vi "Default or Users Font, Leading,Alignment, ASCII or Unicode.vi"(0 "PDF Report":refnum<class "PDF Report Class.lvclass">, 5 "Font":T5={"Name"="", "Size"=-1.0, "Color"=0, "Style"={"Bold"=FALSE, "Italic"=FALSE, "Underline"=FALSE, "Strikeout"=FALSE}, "Type"={"Type&direction"=enum."Select", "Embedded"=FALSE, "Encoding"=""}}, 9 "Paragraphe cluster":T1, 11 "error in (no error)":errorcluster) -> (4 "PDF Report duplicate":refnum<class "PDF Report Class.lvclass">, 6 "Leading":T4=18.0, 8 "Font Ref":refnum<k24>, 10 "Close Font Ref":bool=TRUE, 14 "Aligment":string="JUSTIFY", 15 "error out":errorcluster)   [LabVIEW 2019, in "Exaprom PDF.lvlib"]
doc: "Version 1.0\nDeveloped by Jean-Marc Simard\nCopyright © 2010, Exaprom Inc.\nAll rights reserved.\nLicense: BSD\n\nWith iTextSharp 4.1.6 (http://itextsharp.sourceforge.net)\nunder Mozilla Public License Version 1.1\n(http://www.mozilla.org/MPL/MPL-1.1.html)"
uses:
  LV Class/PDF Report Class/PDF Report Class.lvclass
  Controls/Font Controls/Font complete cluster.ctl
  Controls/Font Controls/Font size.ctl
  Controls/Font Controls/Font color.ctl
  Controls/Font Controls/Type and encoding.ctl
  Controls/Text Controls/Unicode/Type and run direction.ctl
  C:/work/niobrara_lv/labview pdf writer fixing/DLL/itextsharp.dll
  DLL/itextsharp.dll
  Controls/Initialization Controls/Defaut Paragraphe and Line Spacing.ctl
  Controls/Text Controls/Texte alignement.ctl
  Controls/Text Controls/Line spacing.ctl
  Exaprom PDF.lvlib
  LV Class/Fonts Class/Font Class.lvclass
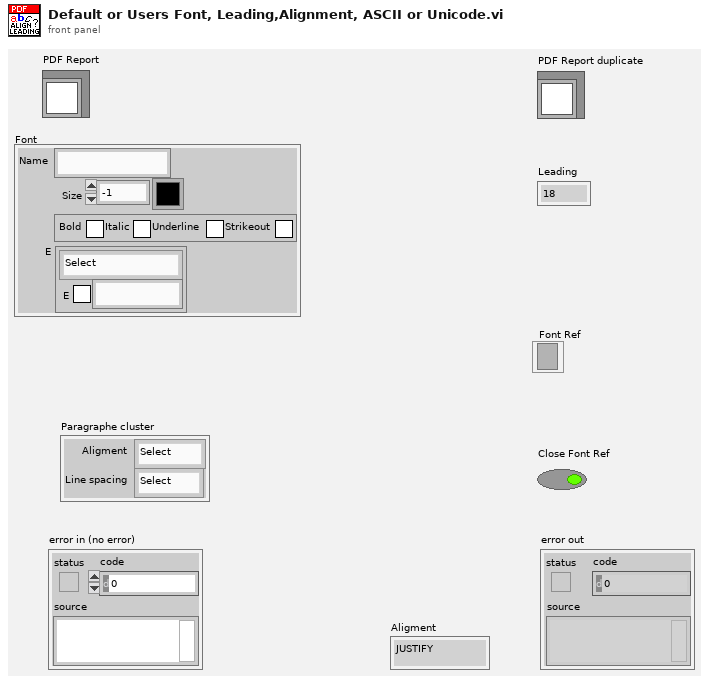
[diagram p1: front panel]
types:
  T1 = typedef "Exaprom PDF.lvlib/Defaut Paragraphe and Line Spacing.ctl" = cluster{" Aligment":T2, "Line spacing":T3}
  T2 = typedef "Exaprom PDF.lvlib/Texte alignement.ctl" = enum16{"Select", "CENTER", "JUSTIFY", "LEFT", "RIGHT"}
  T3 = typedef "Exaprom PDF.lvlib/Line spacing.ctl" = enum16{"Select", "1.0", "1.5", "2.0"}
  T4 = typedef "Exaprom PDF.lvlib/Font size.ctl" = sgl
  T5 = typedef "Exaprom PDF.lvlib/Font complete cluster.ctl" = cluster{"Name":string, "Size":T4, "Color":T6, "Style":cluster{"Bold":bool, "Italic":bool, "Underline":bool, "Strikeout":bool}, "Type":T7}
  T6 = typedef "Exaprom PDF.lvlib/Font color.ctl" = u32
  T7 = typedef "Exaprom PDF.lvlib/Type and encoding.ctl" = cluster{"Type&direction":T8, "Embedded":bool, "Encoding":string}
  T8 = typedef "Exaprom PDF.lvlib/Type and run direction.ctl" = enum16{"Select", "ASCII", "UTF-16", "UTF-16 (default)", "UTF-16 (LTR)", "UTF-16 (RTL)"}
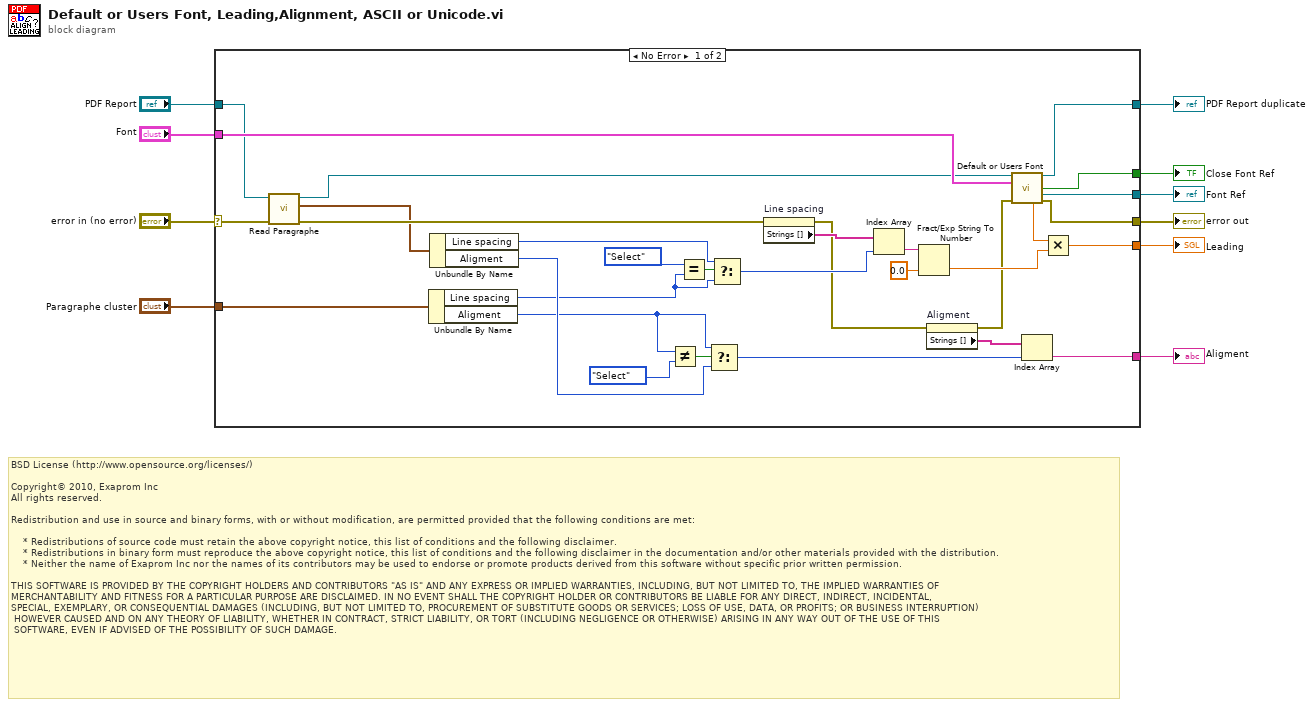
[diagram p0: block diagram]
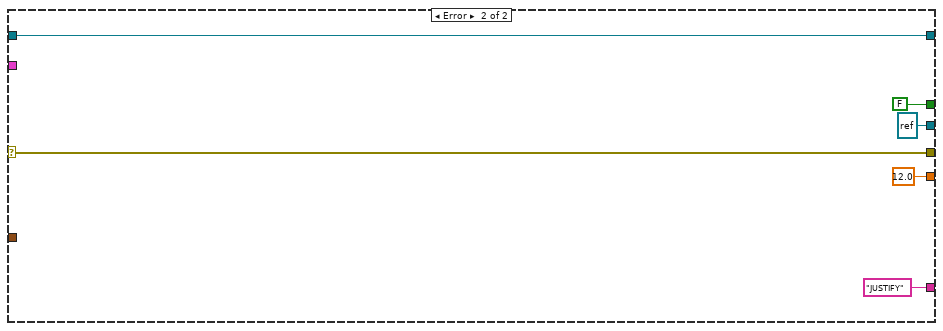
[diagram p2: hidden frame]
diagram:
  # "BSD License (http://www.opensource.org/licenses/)\n\nCopyright© 2010, Exaprom Inc\nAll rights reserved.\n\nRedistribution and use in source and binary forms, with or without modification, are permitted provided that the following conditions are met:\n\n    * Redistributions of source code must retain the above copyright notice, this list of conditions and the following disclaimer.\n    * Redistributions in binary form must reproduce the above copyright notice, this list of conditions and the following disclaimer in the documentation and/or other materials provided with the distribution.\n    * Neither the name of Exaprom Inc nor the names of its contributors may be used to endorse or promote products derived from this software without specific prior written permission.\n\nTHIS SOFTWARE IS PROVIDED BY THE COPYRIGHT HOLDERS AND CONTRIBUTORS \"AS IS\" AND ANY EXPRESS OR IMPLIED WARRANTIES, INCLUDING, BUT NOT LIMITED TO, THE IMPLIED WARRANTIES OF \nMERCHANTABILITY AND FITNESS FOR A PARTICULAR PURPOSE ARE DISCLAIMED. IN NO EVENT SHALL THE COPYRIGHT HOLDER OR CONTRIBUTORS BE LIABLE FOR ANY DIRECT, INDIRECT, INCIDENTAL,\nSPECIAL, EXEMPLARY, OR CONSEQUENTIAL DAMAGES (INCLUDING, BUT NOT LIMITED TO, PROCUREMENT OF SUBSTITUTE GOODS OR SERVICES; LOSS OF USE, DATA, OR PROFITS; OR BUSINESS INTERRUPTION)\n HOWEVER CAUSED AND ON ANY THEORY OF LIABILITY, WHETHER IN CONTRACT, STRICT LIABILITY, OR TORT (INCLUDING NEGLIGENCE OR OTHERWISE) ARISING IN ANY WAY OUT OF THE USE OF THIS\n SOFTWARE, EVEN IF ADVISED OF THE POSSIBILITY OF SUCH DAMAGE."
  n1 = case shown="No Error" "error in (no error)" {
    selector: "error in (no error)" -> [w15 w46]
    tunnel: [w41 "JUSTIFY"] -> w10
    tunnel: "Paragraphe cluster" -> [w40 _]
    tunnel: [w23 T4 12.0 ("Font Size")] -> w8
    tunnel: "PDF Report" -> [w12 w47]
    tunnel: [w22 w47] -> w6
    tunnel: "Font" -> [w21 _]
    tunnel: [w20 FALSE ("Close Font Ref")] -> w4
    tunnel: [w19 refnum<k24> refnum ("Font Ref")] -> w3
    tunnel: [w16 w46] -> w2
    frame No Error {
      n2 = call-dynamic "Read Paragraphe.vi"("error in (no error)"=w15, "PDF Report Class in"=w12) -> ("error out"=w14:errorcluster, "Paragraphe cluster"=w13:T1, "PDF Report Class out"=w11:refnum<class "PDF Report Class.lvclass">)  [unwired: 7 in]
      n3 = Unbundle By Name(w40) -> ("Line spacing"=w30:T3, "Aligment"=w29:T2)
      n4 = Unbundle By Name(w13) -> ("Line spacing"=w32:T3, "Aligment"=w31:T2)
      n5 = Not Equal?(x=w29, y=Texte_alignement."Select" ("Aligment 2")) -> (x != y?=w34:bool)
      n6 = Equal?(x=Line_spacing."Select", y=w30) -> (x = y?=w36:bool)
      n7 = Select(t=w29, s=w34, f=w31) -> (s? t:f=w33:T2)
      n8 = Select(t=w32, s=w36, f=w30) -> (s? t:f=w35:T3)
      n9 = property on="Line spacing" class="Enum (strict)"(error in=w14) -> (error out=w26:errorcluster, "Strings []"=w27:string[])  [unwired: 1 in, 1 out]
      n10 = Index Array(array=w27, index=w35) -> (element=w38:string)
      n11 = Fract/Exp String To Number(string=w38, default (0 dbl)=sgl 0.0 ("default (0 DBL)")) -> (number=w24:sgl)  [unwired: 3 out]
      n12 = property on="Aligment" class="Enum (strict)"(error in=w26) -> (error out=w17:errorcluster, "Strings []"=w25:string[])  [unwired: 1 in, 1 out]
      n13 = call "Default or Users Font.vi"("PDF Report"=w11, "Font"=w21, "error in (no error)"=w17) -> ("PDF Report duplicate"=w22:refnum<class "PDF Report Class.lvclass">, "Close Font Ref"=w20:bool, "Font Ref"=w19:refnum<k24>, "Font Size"=w18:T4, "error out"=w16:errorcluster)  [unwired: 7 in, 1 out]
      n14 = Index Array(array=w25, index=w33) -> (element=w41:string)
      n15 = Multiply(x=w18, y=w24) -> (x*y=w23:T4)
    }
    frame Error {
    }
  }
  "PDF Report duplicate" <- w6
  "error out" <- w2
  "Font Ref" <- w3
  "Leading" <- w8
  "Aligment" <- w10
  "Close Font Ref" <- w4
